vi "DUT properties to string array.vi"(11 "DUT Parameters":T1) -> (2 "Parameter Names":string[](array[string]), 3 "Values (strings)":string[](array[string]))   [LabVIEW 2017]
uses:
  DataTypes/DUT parameters.ctl
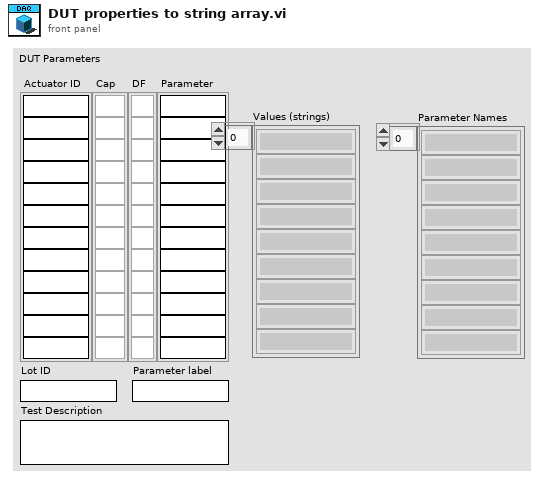
[diagram p1: front panel]
types:
  T1 = typedef "DUT parameters.ctl" = cluster{"Actuator ID":string[], "Cap":dbl[], "DF":dbl[], "Parameter":string[], "Lot ID":string, "Parameter label":string, "Test Description":string}
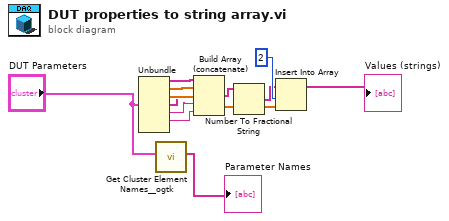
[diagram p0: block diagram]
diagram:
  n1 = Unbundle("DUT Parameters") -> ("Actuator ID"=w2:string[], "Cap"=w1:dbl[], "DF"=w9:dbl[], "Parameter"=w3:string[], "Lot ID"=w4:string, "Parameter label"=w5:string)  [unwired: 1 out]
  n2 = call <userlib>:"Get Cluster Element Names__ogtk.vi"("Cluster"="DUT Parameters") -> ("Element Names"=→"Parameter Names":string[])  [unwired: 9 in, 1 out]
  n3 = Build Array (concatenate)(w2, w1, w3, w4, w5) -> (w6:string[])
  n4 = Number To Fractional String(number=w6) -> (F-format string=w7:string[])  [unwired: 3 in]
  n5 = Insert Into Array(array=w7, index=2, new element=w9) -> (→"Values (strings)":string[])
